vi "Test SPIVI.vi"() -> ()   [LabVIEW 2016]
uses:
  Typedefs/SPI Configuration.ctl
  SubVIs/U8 Array Reverse Bit Order.vi
  SPIVI.lvlib
panel:
  in  "Sample Rate":dbl=10000000.0 format="%#_13p"
  in  "Reverse Bit Order":bool
  in  "MOSI Data":u8[](array[numeric]) format="%x"
  in  "Stop Button":bool
  out "SPI Signals":digitalwaveform(graph)
  out "MISO Data":u8[](array[numeric]) format="%x"
  in  "SPI Configuration":T1={"CLK Frequency (Hz)"=250000, "CPOL"=FALSE, "CPHA"=FALSE, "CS Channel"="PXI1Slot3/port0/line3", "CLK Channel"="PXI1Slot3/port0/line0", "MOSI Channel"="PXI1Slot3/port0/line1", "MISO Channel"="PXI1Slot3/port0/line2", "Active CS"=FALSE, "Dig In Task"="", "Dig Out Task"=""} {"CLK Frequency (Hz)" format="%#.6p"}
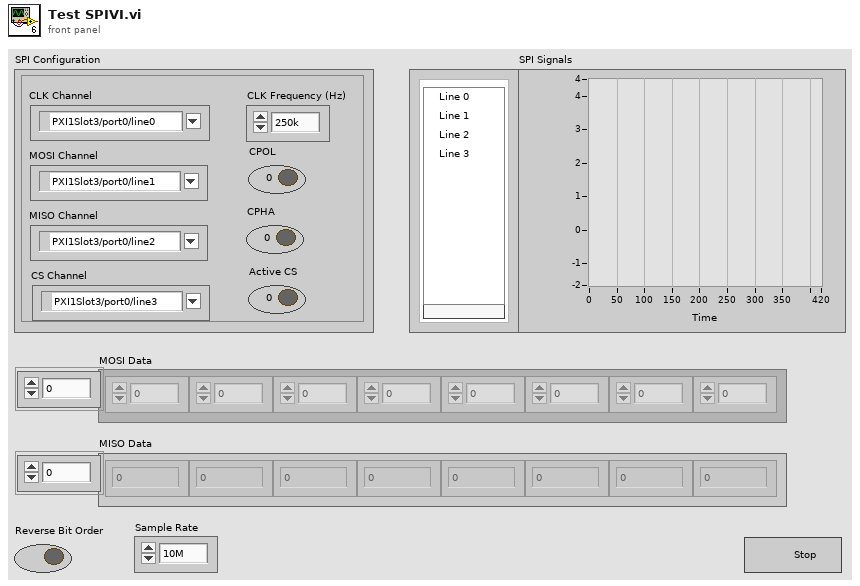
[diagram p1: front panel]
types:
  T1 = typedef "SPIVI.lvlib/SPI Configuration.ctl" = cluster{"CLK Frequency (Hz)":u32, "CPOL":bool, "CPHA":bool, "CS Channel":tag, "CLK Channel":tag, "MOSI Channel":tag, "MISO Channel":tag, "Active CS":bool, "Dig In Task":refnum<k21>, "Dig Out Task":refnum<k21>}
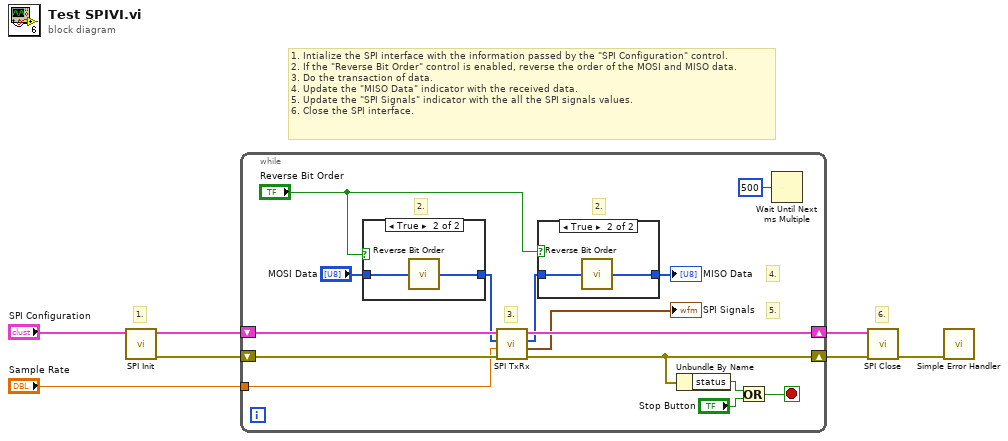
[diagram p0: block diagram]
diagram:
  # "6."
  # "1. Intialize the SPI interface with the information passed by the \"SPI Configuration\" control.\n2. If the \"Reverse Bit Order\" control is enabled, reverse the order of the MOSI and MISO data.\n3. Do the transaction of data.\n4. Update the \"MISO Data\" indicator with the received data.\n5. Update the \"SPI Signals\" indicator with the all the SPI signals values.\n6. Close the SPI interface."
  # "1."
  n1 = call "SPI Init.vi"("SPI Configuration In"="SPI Configuration") -> ("Error Out"=w6:errorcluster, "SPI Configuration Out"=w7:T1)  [unwired: 9 in]
  n2 = while {
    shift-right: [w19] -> w5
    shift-left: w7 -> [w22]
    shift-right: [w14] -> w4
    shift-left: w6 -> [w21]
    tunnel: "Sample Rate" -> [w8]
    stop <- w17 stop-if-true
    # "5."
    # "4."
    # "3."
    # "2."
    # "2."
    n3 = case shown="True" "Reverse Bit Order" {
      tunnel: "MOSI Data" -> [w26 w28]
      tunnel: [w26 w27] -> w12
      frame False {
      }
      frame True {
        n4 = call-poly "Reverse Bit Order.vi"("U8 Array Data In"=w28) -> ("U8 Array Data Out"=w27:u8[])
      }
    }
    n5 = call "SPI TxRx.vi"("Error In"=w21, "Sample Rate"=w8, "MOSI Data"=w12, "SPI Configuration In"=w22) -> ("Error Out"=w14:errorcluster, "SPI Signals"=→"SPI Signals":digitalwaveform, "MISO Data"=w10:u8[], "SPI Configuration Out"=w19:T1)  [unwired: 4 in]
    n6 = case shown="True" "Reverse Bit Order" {
      tunnel: [w23 w25] -> w11
      tunnel: w10 -> [w23 w24]
      frame False {
      }
      frame True {
        n7 = call-poly "Reverse Bit Order.vi"("U8 Array Data In"=w24) -> ("U8 Array Data Out"=w25:u8[])
      }
    }
    "MISO Data" <- w11
    n8 = Unbundle By Name(w14) -> ("status"=w20:bool)
    n9 = Or(x=w20, y="Stop Button") -> (x .or. y?=w17:bool)
    n10 = Wait Until Next ms Multiple(millisecond multiple=u32 500) -> ()  [unwired: 1 out]
  }
  n11 = call "SPI Close.vi"("Error In"=w4, "SPI Configuration In"=w5) -> ("Error Out"=w2:errorcluster)  [unwired: 8 in, 1 out]
  n12 = call <vilib>:"Simple Error Handler.vi"("error in (no error)"=w2) -> ()  [unwired: 4 in, 5 out]
